vi "Text Description.vi"(11 "Send in":refnum<class "Send.lvclass">) -> (2 "Description":string, 3 "Send out":refnum<class "Send.lvclass">)   [LabVIEW 2011, in "Messenging.lvlib" / "Send.lvclass"]
uses:
  Send.lvclass
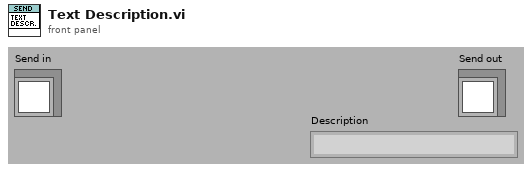
[diagram p1: front panel]
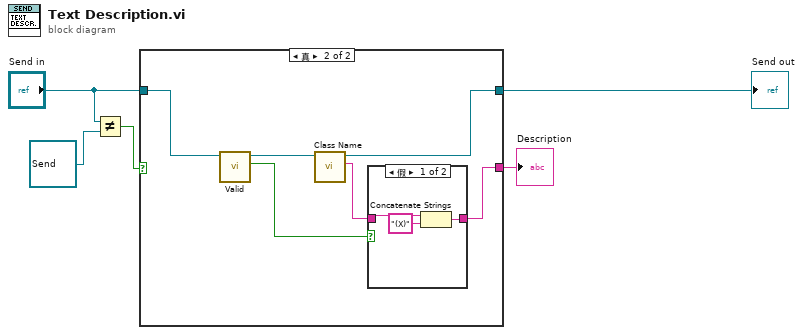
[diagram p0: block diagram]
diagram:
  n1 = Not Equal?(x="Send in", y=refnum<class "Send.lvclass"> refnum ("Send in")) -> (x != y?=w1:bool)
  n2 = case shown="真" w1 {
    tunnel: [w6 w12] -> w5
    tunnel: [_ w8] -> w4
    tunnel: "Send in" -> [w6 w10]
    frame False {
    }
    frame True {
      n3 = call-dynamic "Valid.vi"("Send in"=w10) -> ("Valid?"=w9:bool, "Send out"=w11:refnum<class "Send.lvclass">)  [unwired: 9 out]
      n4 = call "Class Name.vi"("Send in"=w11) -> ("Class Name"=w7:string, "Send out"=w12:refnum<class "Send.lvclass">)  [unwired: 1 in, 8 out]
      n5 = case shown="假" w9 {
        tunnel: [w15 w16] -> w8
        tunnel: w7 -> [w14 w16]
        frame False {
          n6 = Concatenate Strings(w14, "(X)" ("string")) -> (w15:string)
        }
        frame True {
        }
      }
    }
  }
  "Send out" <- w5
  "Description" <- w4
